vi "Periodic Tasks.vi"(8 "error in":errorcluster) -> ()   [LabVIEW 2015]
doc: "This VI runs in parallel to other tasks. It can contain as many user-defined periodic loops as you need. These can carry out PID or other sorts of timed response."
uses:
  Common Code/Change Detect Int.vi
  Robot Global Data.vi
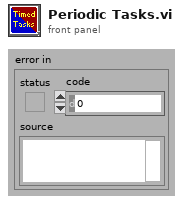
[diagram p1: front panel]
types:
  T1 = typedef "WPI_DriverStationRobotMode2.ctl" = enum16{"Autonomous Disabled", "Autonomous Enabled", "Teleop Disabled", "Teleop Enabled", "Disconnected", "Finish", "Test Disabled", "Test Enabled", "Emergency Stopped"}
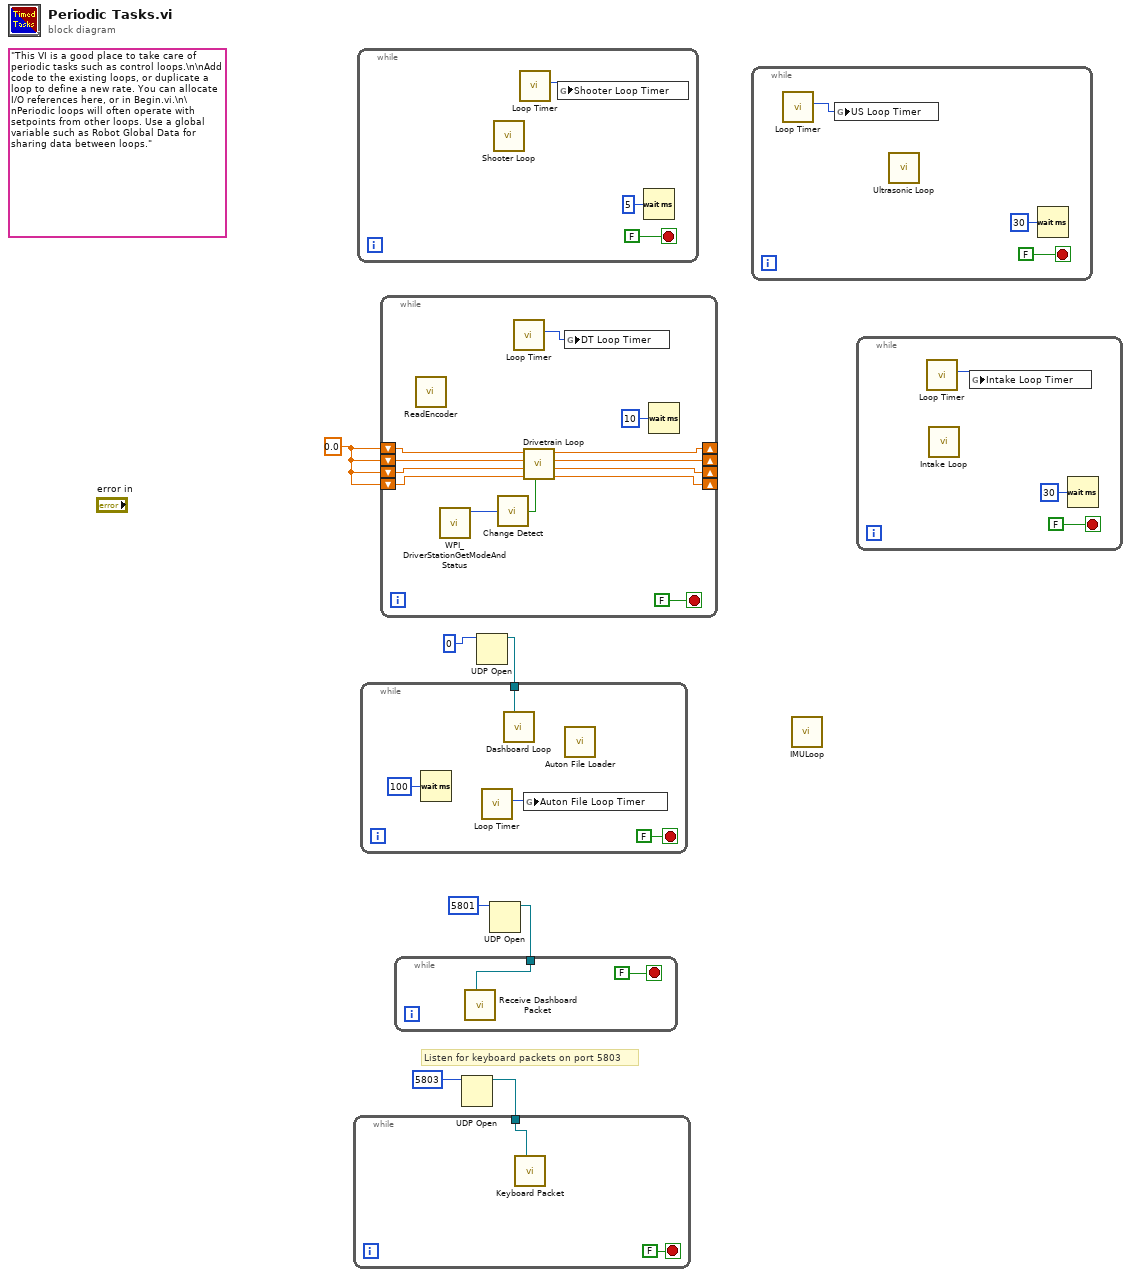
[diagram p0: block diagram]
diagram:
  w1 = 0.0 ("Timer 1 out")
  (unwired) "This VI is a good place to take care of periodic tasks such as control loops.\n\nAdd code to the existing loops, or duplicate a loop to define a new rate. You can allocate I/O references here, or in Begin.vi.\n\nPeriodic loops will often operate with setpoints from other loops. Use a global variable such as Robot Global Data for sharing data between loops."
  # "Listen for keyboard packets on port 5803"
  n1 = while {
    stop <- FALSE stop-if-true
    n2 = call "Shooter Loop.vi"() -> ()  [unwired: 12 in]
    n3 = call "Loop Timer.vi"() -> ("dt"=w8:u32)  [unwired: 11 in]
    n4 = global write "Robot Global Data.vi" "Shooter Loop Timer"(w8) -> ()
    n5 = Wait (ms)(milliseconds to wait=u32 5) -> ()  [unwired: 1 out]
  }
  n6 = while {
    shift-right: [w15] -> _
    shift-left: w1 -> [w16]
    shift-right: [w19] -> _
    shift-left: w1 -> [w20]
    shift-right: [w14] -> _
    shift-left: w1 -> [w18]
    shift-right: [w13] -> _
    shift-left: w1 -> [w17]
    stop <- FALSE stop-if-true
    n7 = call "ReadEncoder.vi"() -> ()  [unwired: 11 in, 1 out]
    n8 = call <vilib>:"WPI_DriverStationGetModeAndStatus.vi"() -> ("Robot Mode"=w21:T1)  [unwired: 10 in, 1 out]
    n9 = call-poly "Change Detect.vi"("In"=w21) -> ("Changed?"=w12:bool)
    n10 = call "Loop Timer.vi"() -> ("dt"=w11:u32)  [unwired: 11 in]
    n11 = call "Drivetrain Loop.vi"("Reset the clock"=w12, "In 4"=w17, "In 3"=w18, "In 2"=w20, "In 1"=w16) -> ("Out 4"=w13:dbl, "Out 3"=w14:dbl, "Out 2"=w19:dbl, "Out 1"=w15:dbl)  [unwired: 3 in]
    n12 = global write "Robot Global Data.vi" "DT Loop Timer"(w11) -> ()
    n13 = Wait (ms)(milliseconds to wait=u32 10) -> ()  [unwired: 1 out]
  }
  n14 = UDP Open(11:u16 5803 ("port")) -> (port=w2:refnum<k16>)  [unwired: 4 in, 2 out]
  n15 = while {
    tunnel: w2 -> [w24]
    stop <- FALSE stop-if-true
    n16 = call "Keyboard Packet.vi"("connection ID"=w24) -> ()  [unwired: 11 in]
  }
  n17 = UDP Open(11:0) -> (port=w5:refnum<k16>)  [unwired: 4 in, 2 out]
  n18 = while {
    tunnel: w5 -> [w27]
    stop <- FALSE stop-if-true
    n19 = Wait (ms)(milliseconds to wait=u32 100) -> ()  [unwired: 1 out]
    n20 = call "Loop Timer.vi"() -> ("dt"=w26:u32)  [unwired: 11 in]
    n21 = call "Dashboard Loop.VI"("connection ID"=w27) -> ()  [unwired: 11 in]
    n22 = global write "Robot Global Data.vi" "Auton File Loop Timer"(w26) -> ()
    n23 = call "Auton File Loader.vi"() -> ()  [unwired: 12 in]
  }
  n24 = UDP Open(11:u16 5801 ("port")) -> (port=w7:refnum<k16>)  [unwired: 4 in, 2 out]
  n25 = while {
    tunnel: w7 -> [w30]
    stop <- FALSE stop-if-true
    n26 = call "Receive Dashboard Packet.vi"("connection ID"=w30) -> ()  [unwired: 11 in]
  }
  n27 = while {
    stop <- FALSE stop-if-true
    n28 = call "Loop Timer.vi"() -> ("dt"=w32:u32)  [unwired: 11 in]
    n29 = global write "Robot Global Data.vi" "US Loop Timer"(w32) -> ()
    n30 = call "Ultrasonic Loop.vi"() -> ()  [unwired: 12 in]
    n31 = Wait (ms)(milliseconds to wait=u32 30) -> ()  [unwired: 1 out]
  }
  n32 = call "IMULoop.vi"() -> ()  [unwired: 12 in]
  n33 = while {
    stop <- FALSE stop-if-true
    n34 = call "Loop Timer.vi"() -> ("dt"=w35:u32)  [unwired: 11 in]
    n35 = call "Intake Loop.vi"() -> ()  [unwired: 12 in]
    n36 = global write "Robot Global Data.vi" "Intake Loop Timer"(w35) -> ()
    n37 = Wait (ms)(milliseconds to wait=u32 30) -> ()  [unwired: 1 out]
  }
